vi "SWERVE_DRIVE_ACQUIRE.vi"(6 "Pass_Through_Time":dbl=-1.0 format="%33.4f", 8 "error in":errorcluster) -> (0 "error out":errorcluster)   [LabVIEW 2023]
uses:
  <vilib>/Rock Robotics/WPI/DriverStation/WPI_DriverStationRobotMode2.ctl
  <vilib>/Rock Robotics/WPI/ThirdParty/JAS_Junk/TrajLib/TypeDef/ROTATION2D.ctl
  <vilib>/Rock Robotics/WPI/ThirdParty/JAS_Junk/TrajLib/MathUtil_InputModulus.vi
  <vilib>/Rock Robotics/WPI/ThirdParty/JAS_Junk/TrajLib/Translation2d_Create.vi
  SWERVE_DRIVE_GLOBALS.vi
  Robot Global Data.vi
  <vilib>/Rock Robotics/WPI/Utilities/WPI_GetSetVariantRefNum.vi
  <vilib>/Rock Robotics/Network Tables/NT Write Number.vi
  <vilib>/Rock Robotics/WPI/ThirdParty/Phoenix-LabVIEW/Pigeon IMU/CTRE_PigeonIMU_GetYPR.vi
  <vilib>/Rock Robotics/Network Tables/NT Read Numeric Array.vi
  <vilib>/Rock Robotics/Network Tables/NT Write Boolean.vi
  <vilib>/Rock Robotics/Network Tables/NT Read Boolean.vi
  <vilib>/Rock Robotics/WPI/ThirdParty/JAS_Junk/TrajLib/Trajectory_Library.lvlib
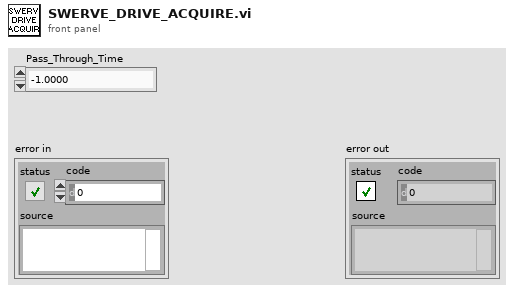
[diagram p1: front panel]
types:
  T1 = typedef "WPI_DriverStationRobotMode2.ctl" = enum16{"Autonomous Disabled", "Autonomous Enabled", "Teleop Disabled", "Teleop Enabled", "Disconnected", "Finish", "Test Disabled", "Test Enabled", "Emergency Stopped"}
  T2 = typedef "Trajectory_Library.lvlib/ROTATION2D.ctl" = cluster{"VALUE":dbl, "COS":dbl, "SIN":dbl}
  T3 = enum16{"Talon FX, P5", "Talon FX, P6", "SPARK MAX"}
  T4 = typedef "Trajectory_Library.lvlib/SWERVE_DRIVE_MODULE_POSITION.ctl" = cluster{"Distance":dbl, "Angle":T2, "P":bool}
  T5 = typedef "Trajectory_Library.lvlib/SWERVE_DRIVE_MODULE_STATE.ctl" = cluster{"Speed":dbl, "Angle":T2}
  T6 = typedef "CTRE_PigeonIMU_DeviceRef.ctl" = cluster{"DeviceStatus":errorcluster, "Device Number":u8, "Type":T7, "Device ID":u32, "Handle":u64, "UsageFrame":u32, "Library Path":path}
  T7 = typedef "CTRE_PigeonIMU_ConnectionType.ctl" = u32
  T8 = typedef "Trajectory_Library.lvlib/SWERVE_DRIVE_KINEMATICS.ctl" = cluster{"NumModules":i32, "InverseKinematics":T9, "ForwardKinematics":T9, "Modules":T10[], "PrevCoR":T10, "SavedModuleStates":T5[]}
  T9 = typedef "NI_Matrix.lvlib/RealMatrix.ctl" = dbl[][]
  T10 = typedef "Trajectory_Library.lvlib/TRANSLATION2D.ctl" = cluster{"X":dbl, "Y":dbl}
  T11 = typedef "Trajectory_Library.lvlib/CHASSIS_SPEEDS.ctl" = cluster{"vX":dbl, "vY":dbl, "vOmega":dbl}
  T12 = typedef "WPI_JoystickDevRef.ctl" = cluster{"Device":T13}
  T13 = typedef "WPI_JoystickDeviceEnum.ctl" = enum16{"USB 0", "USB 1", "USB 2", "USB 3", "USB 4", "USB 5"}
  T14 = typedef "Trajectory_Library.lvlib/POSE2D.ctl" = cluster{"TRANSLATION":T10, "ROTATION":T2}
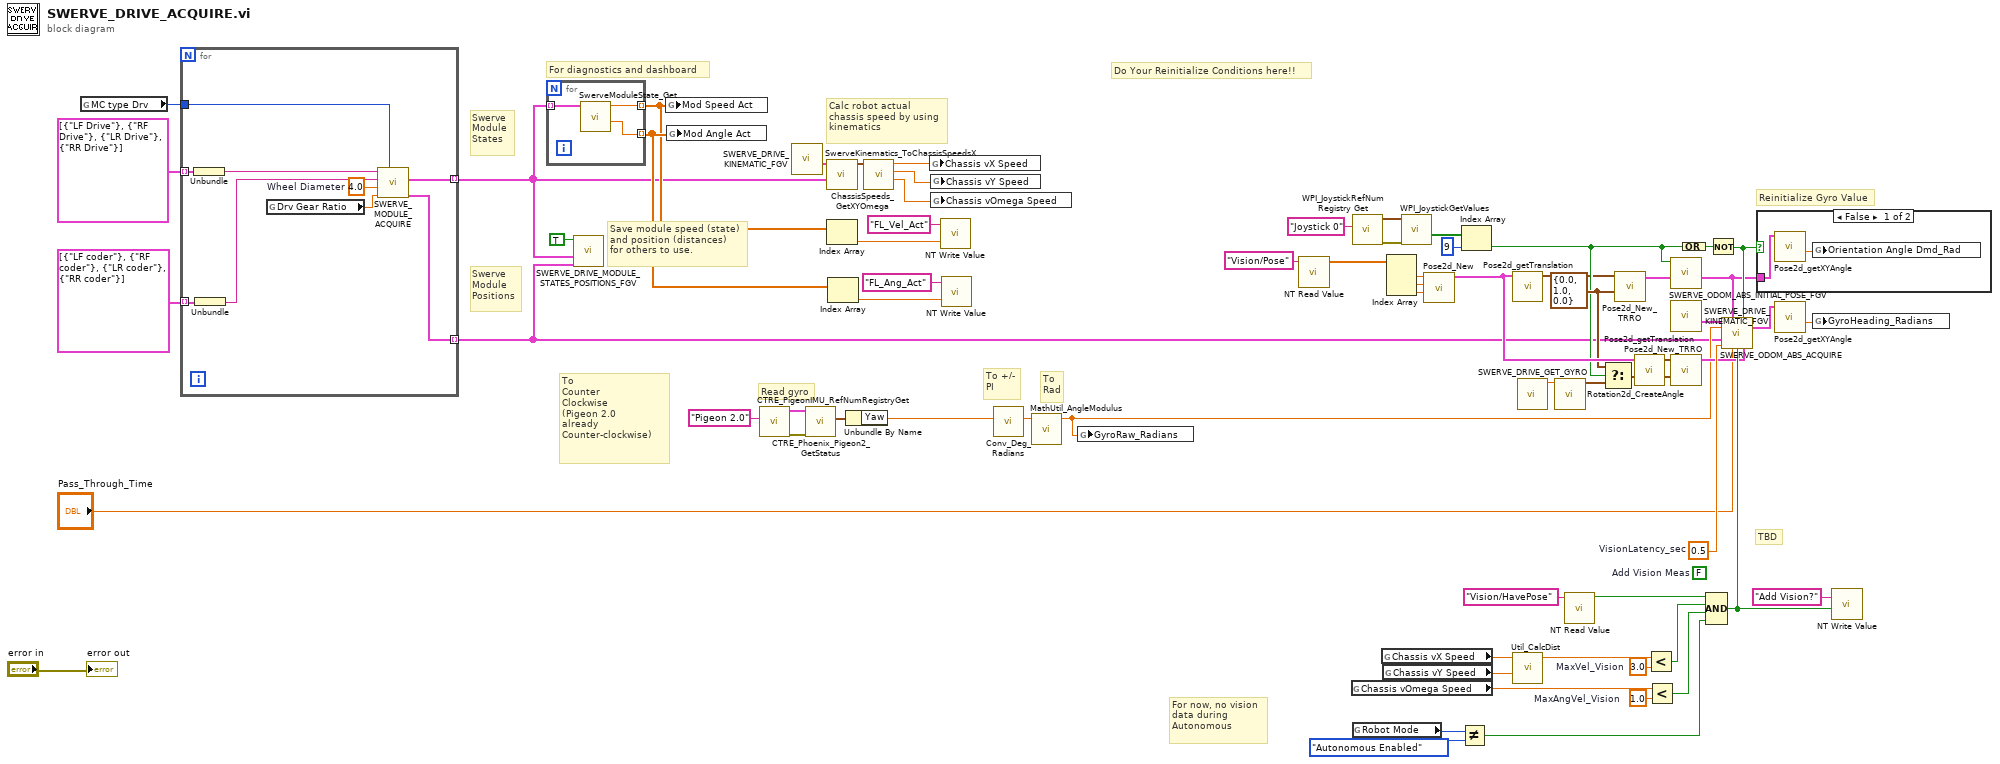
[diagram p0: block diagram]
diagram:
  w51 = 1.0  # MaxAngVel_Vision
  w62 = 0.5  # VisionLatency_sec
  w47 = 3.0  # MaxVel_Vision
  w43 = T2 {"VALUE"=0.0, "COS"=1.0, "SIN"=0.0} ("ROTATION")
  (unwired) FALSE  # Add Vision Meas
  # "TBD"
  # "For now, no vision data during Autonomous"
  # "Reinitialize Gyro Value"
  # "Do Your Reinitialize Conditions here!!"
  # "Swerve\nModule\nStates"
  # "Save module speed (state)\nand position (distances)\nfor others to use."
  # "Swerve\nModule\nPositions"
  # "For diagnostics and dashboard"
  # "Calc robot actual\nchassis speed by using\nkinematics"
  # "To\nCounter\nClockwise\n(Pigeon 2.0\nalready \nCounter-clockwise)"
  # "To +/-\nPI"
  # "To\nRad"
  # "Read gyro"
  n1 = global read "SWERVE_DRIVE_GLOBALS.vi" "MC type Drv"() -> (w20:T3)
  n2 = for {
    tunnel: [w73] -> w15 mode=indexing
    tunnel: [w74] -> w14 mode=indexing
    tunnel: cluster{string}[] [{"LF coder"}, {"RF coder"}, {"LR coder"}, {"RR coder"}] ("CANcoder ref") -> [w77] mode=indexing
    tunnel: cluster{string}[] [{"LF Drive"}, {"RF Drive"}, {"LR Drive"}, {"RR Drive"}] ("Drive ref") -> [w76] mode=indexing
    tunnel: w20 -> [w75]
    w69 = 4.0  # Wheel Diameter
    n3 = Unbundle(w76) -> (w72:string)
    n4 = Unbundle(w77) -> (w71:string)
    n5 = global read "SWERVE_DRIVE_GLOBALS.vi" "Drv Gear Ratio"() -> (w70:dbl)
    n6 = call "SWERVE_MODULE_ACQUIRE.vi"("MC type Drv"=w75, "Drv Gear Ratio"=w70, "Wheel Diameter IN"=w69, "Encoder Name"=w71, "Drive Motor Name"=w72) -> ("SWERVE_DRIVE_MODULE_POSITION"=w73:T4, "SWERVE_DRIVE_MODULE_STATE"=w74:T5)  [unwired: 5 in]
  }
  n7 = for {
    tunnel: w14 -> [w80] mode=indexing
    tunnel: [w78] -> w26 mode=indexing
    tunnel: [w79] -> w22 mode=indexing
    n8 = call <vilib>:"SwerveModuleState_Get.vi"("Desired State"=w80) -> ("Angle RADIANS"=w78:dbl, "Speed M/S"=w79:dbl)  [unwired: 9 in]
  }
  n9 = call "SWERVE_DRIVE_MODULE_STATES_POSITIONS_FGV.vi"("in Current Module Positions"=w15, "in Current Module States"=w14, "WRITE"=TRUE) -> ()  [unwired: 7 in, 2 out]
  n10 = global write "SWERVE_DRIVE_GLOBALS.vi" "Mod Speed Act"(w22) -> ()
  n11 = global write "SWERVE_DRIVE_GLOBALS.vi" "Mod Angle Act"(w26) -> ()
  n12 = call <vilib>:"CTRE_PigeonIMU_RefNumRegistryGet.vi"("refnum name"="Pigeon 2.0") -> ("error out"=w4:errorcluster, "PigeonIMUDevRef"=w5:T6)  [unwired: 9 in]
  n13 = call "SWERVE_DRIVE_KINEMATIC_FGV.vi"() -> ("out SWERVE_DRIVE_KINEMATICS"=w8:T8)  [unwired: 11 in]
  n14 = call-poly <vilib>:"CTRE_Phoenix_Pigeon2_GetStatus.vi"("error in (no error)"=w4, "PigeonIMUDevRef"=w5) -> ("Yaw Pitch Roll"=w6:cluster{"Yaw":dbl, "Pitch":dbl, "Roll":dbl})  [unwired: 7 in, 2 out]
  n15 = call <vilib>:"SwerveKinematics_ToChassisSpeedsX.vi"("WheelStates"=w14, "in SWERVE_DRIVE_KINEMATICS"=w8) -> ("Chassis Speed"=w19:T11)  [unwired: 9 in]
  n16 = Index Array(array=w22) -> (element=w21:dbl)  [unwired: 1 in]
  n17 = Index Array(array=w26) -> (element=w24:dbl)  [unwired: 1 in]
  n18 = Unbundle By Name(w6) -> ("Yaw"=w10:dbl)
  n19 = call <vilib>:"ChassisSpeeds_GetXYOmega.vi"("CHASSIS"=w19) -> ("vAngular"=w18:dbl, "vY"=w17:dbl, "vX"=w16:dbl)  [unwired: 8 in]
  n20 = global write "SWERVE_DRIVE_GLOBALS.vi" "Chassis vX Speed"(w16) -> ()
  n21 = global write "SWERVE_DRIVE_GLOBALS.vi" "Chassis vY Speed"(w17) -> ()
  n22 = global write "SWERVE_DRIVE_GLOBALS.vi" "Chassis vOmega Speed"(w18) -> ()
  n23 = call-poly <vilib>:"NT Write Value.vi"("value"=w21, "name"="FL_Vel_Act") -> ()  [unwired: 9 in, 1 out]
  n24 = call-poly <vilib>:"NT Write Value.vi"("value"=w24, "name"="FL_Ang_Act") -> ()  [unwired: 9 in, 1 out]
  n25 = call <vilib>:"Conv_Deg_Radians.vi"("Degress"=w10) -> ("Radians"=w9:dbl)  [unwired: 10 in]
  n26 = call <vilib>:"MathUtil_AngleModulus.vi"("InputAngle"=w9) -> ("ModulsAngle"=w38:dbl)  [unwired: 10 in]
  n27 = global write "SWERVE_DRIVE_GLOBALS.vi" "GyroRaw_Radians"(w38) -> ()
  n28 = call-poly <vilib>:"NT Read Value.vi"("name"="Vision/Pose") -> ("value"=w53:dbl[])  [unwired: 8 in, 2 out]
  n29 = global read "SWERVE_DRIVE_GLOBALS.vi" "Chassis vOmega Speed"() -> (w65:dbl)
  n30 = call <vilib>:"WPI_JoystickRefNum Registry Get.vi"("refnum name"="Joystick 0") -> ("error out"=w27:errorcluster, "JoystickDevRef"=w29:T12)  [unwired: 1 in, 8 out]
  n31 = global read "Robot Global Data.vi" "Robot Mode"() -> (w66:T1)
  n32 = global read "SWERVE_DRIVE_GLOBALS.vi" "Chassis vX Speed"() -> (w63:dbl)
  n33 = global read "SWERVE_DRIVE_GLOBALS.vi" "Chassis vY Speed"() -> (w64:dbl)
  n34 = Index Array(array=w53) -> (element #1=w54:dbl, element #2=w55:dbl, element #3=w56:dbl)  [unwired: 3 in]
  n35 = call <vilib>:"WPI_JoystickGetValues.vi"("error in (no error)"=w27, "JoystickDevRef"=w29) -> ("Buttons"=w28:bool[])  [unwired: 5 in, 4 out]
  n36 = call <vilib>:"Pose2d_New.vi"("Heading"=w56, "Y"=w55, "X"=w54) -> ("out POSe"=w57:T14)  [unwired: 8 in]
  n37 = Not Equal?(x=w66, y=WPI_DriverStationRobotMode2."Autonomous Enabled") -> (x != y?=w68:bool)
  n38 = Index Array(array=w28, index=9) -> (element=w42:bool)
  n39 = call <vilib>:"Pose2d_getTranslation.vi"("in POSE"=w57) -> ("outTRANSLATION"=w37:T10)  [unwired: 10 in]
  n40 = call <vilib>:"Util_CalcDist.vi"("Y"=w64, "X"=w63) -> ("DIST"=w50:dbl)  [unwired: 9 in]
  n41 = call "SWERVE_DRIVE_GET_GYRO.vi"() -> ("Gyro Heading Radians"=w40:dbl)  [unwired: 11 in]
  n42 = call <vilib>:"Rotation2d_CreateAngle.vi"("Angle"=w40) -> ("ROTATION"=w41:T2)  [unwired: 10 in]
  n43 = call-poly <vilib>:"NT Read Value.vi"("name"="Vision/HavePose") -> ("value"=w61:bool)  [unwired: 8 in, 2 out]
  n44 = Select(t=w43, s=w42, f=w41) -> (s? t:f=w44:T2)
  n45 = call <vilib>:"Pose2d_New_TRRO.vi"("ROTATION"=w43, "TRANSLATION"=w37) -> ("outPOSE"=w39:T14)  [unwired: 9 in]
  n46 = call <vilib>:"Pose2d_getTranslation.vi"("in POSE"=w57) -> ("outTRANSLATION"=w45:T10)  [unwired: 10 in]
  n47 = Less?(x=w50, y=w47) -> (x < y?=w48:bool)
  n48 = Less?(x=w65, y=w51) -> (x < y?=w49:bool)
  n49 = call "SWERVE_ODOM_ABS_INITIAL_POSE_FGV.vi"("in INITIAL_POSE2D"=w39, "WRITE"=w42) -> ("out INITIAL_POSE2D"=w33:T14)  [unwired: 9 in]
  n50 = call "SWERVE_DRIVE_KINEMATIC_FGV.vi"() -> ("out SWERVE_DRIVE_KINEMATICS"=w11:T8)  [unwired: 11 in]
  n51 = call <vilib>:"Pose2d_New_TRRO.vi"("ROTATION"=w44, "TRANSLATION"=w45) -> ("outPOSE"=w46:T14)  [unwired: 9 in]
  n52 = Compound Arithmetic op=OR(w42) -> (w32:bool)
  n53 = Compound Arithmetic op=AND(w61, w48, w49, w68) -> (w58:bool)
  n54 = Not(x=w32) -> (.not. x?=w34:bool)
  n55 = call "SWERVE_ODOM_ABS_ACQUIRE.vi"("in SWERVE_DRIVE_KINEMATICS"=w11, "InitialPose"=w33, "Game Started"=w34, "Gyro_Raw_Rad"=w38, "in Swerve Module Positions"=w15, "VisionLatency_sec"=w62, "Pass_Through_Time"="Pass_Through_Time", "Add Vision Meas"=w58, "visionRobotPose"=w46) -> ("ODOM_POSE"=w35:T14)  [unwired: 5 in, 1 out]
  n56 = case shown="False" w34 {
    tunnel: w33 -> [w82 _]
    frame False {
      n57 = call <vilib>:"Pose2d_getXYAngle.vi"("in POSE"=w82) -> ("Angle"=w81:dbl)  [unwired: 8 in, 2 out]
      n58 = global write "SWERVE_DRIVE_GLOBALS.vi" "Orientation Angle Dmd_Rad"(w81) -> ()
    }
    frame True {
    }
  }
  n59 = call <vilib>:"Pose2d_getXYAngle.vi"("in POSE"=w35) -> ("Angle"=w36:dbl)  [unwired: 8 in, 2 out]
  n60 = global write "SWERVE_DRIVE_GLOBALS.vi" "GyroHeading_Radians"(w36) -> ()
  n61 = call-poly <vilib>:"NT Write Value.vi"("value"=w58, "name"="Add Vision?") -> ()  [unwired: 9 in, 1 out]
  "error out" <- "error in"
